vi "1DSGLToString.vi"(0 "Array":sgl[](array[numeric]), 5 "Precision":i16=6 caption="Precision (6)", 7 "Radix point":T1=enum."Comma (,)" caption="Radix point (,)", 9 "Remove trailing zeroes?":bool=TRUE caption="Remove trailing zeroes? (T)", 11 "Error in":errorcluster caption="Error in (no error)") -> (4 "String":string, 15 "Error out":errorcluster)   [LabVIEW 2017, in "GPString.lvlib"]
doc: "Converts <B>Array</B> to <B>String</B> observing the specified <B>Precision</B> and <B>Radix point</B>.\n\n<B>Radix point</B> can be either: System (localized), period (.), or comma (,).\n\nBy default this VI removes trailing zeroes in the fractional parts. Set <B>Remove trailing zeroes?</B> to False if you want to keep <B>Precision</B> number of digits in the fractional parts, even when the rightmost fractional digits are zeroes.\n\nThis VI is inlined and it runs only if there is no error on <B>Error in</B>.\n\nSteen Schmidt\nGPower\n15/6 2016"
uses:
  GPString.lvlib
  Typedefs/RadixPoint.ctl
panel:
  # "Copyright © 2016\nGPower\nSee enclosed license file for terms and conditions"
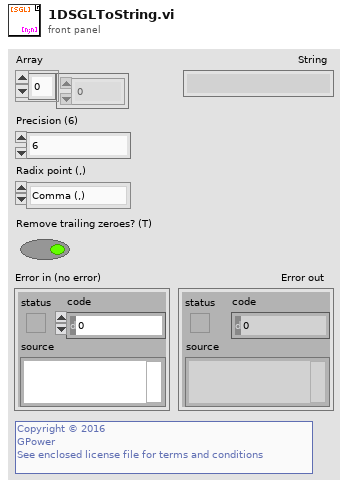
[diagram p1: front panel]
types:
  T1 = typedef "GPString.lvlib/RadixPoint.ctl" = enum16{"System", "Period (.)", "Comma (,)"}
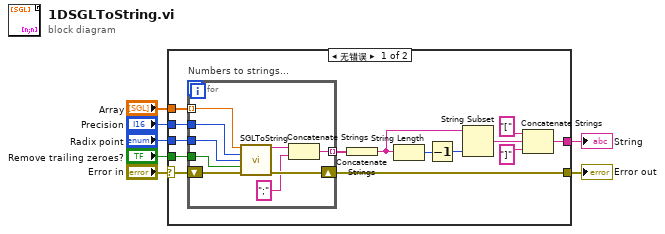
[diagram p0: block diagram]
diagram:
  n1 = case shown="无错误" "Error in" {
    selector: "Error in" -> [w14 w31]
    tunnel: "Array" -> [w21 _]
    tunnel: "Radix point" -> [w12 _]
    tunnel: "Precision" -> [w20 _]
    tunnel: [w16 _] -> w4
    tunnel: [w15 w31] -> w3
    tunnel: "Remove trailing zeroes?" -> [w13 _]
    frame No Error {
      n2 = for "Numbers to strings..." {
        tunnel: w21 -> [w30] mode=indexing
        shift-right: [w26] -> w15
        shift-left: w14 -> [w29]
        tunnel: w12 -> [w28]
        tunnel: w20 -> [w27]
        tunnel: [w24] -> w19 mode=indexing
        tunnel: w13 -> [w23]
        n3 = call "SGLToString.vi"("Number"=w30, "Precision"=w27, "Radix point"=w28, "Remove trailing zeroes?"=w23, "Error in"=w29) -> ("String"=w25:string, "Error out"=w26:errorcluster)  [unwired: 9 in]
        n4 = Concatenate Strings(w25, ";" ("Secondary separator char")) -> (w24:string)
      }
      n5 = Concatenate Strings(w19) -> (w11:string)
      n6 = String Length(string=w11) -> (length=w9:i32)
      n7 = Decrement(x=w9) -> (x-1=w10:i32)
      n8 = String Subset(string=w11, length (rest)=w10) -> (substring=w8:string)  [unwired: 1 in]
      n9 = Concatenate Strings("[" ("substring"), w8, "]" ("substring")) -> (w16:string)
    }
    frame Error {
    }
  }
  "String" <- w4
  "Error out" <- w3
